vi "AH 2700 Single Measurement.vi"() -> ()   [LabVIEW 2019]
doc: "This example shows how to configure the bridge, take a single capacitance measurement, read the results from the bridge, and parse the measurement results."
uses:
  Andeen-Hagerling 2700(400 firmware).lvlib
panel:
  out "Loss Greater Than":string
  out "Attentap":string
  out "Sample Switch":i32
  out "Frequency (Hz)":dbl
  out "Result Units":i32(ring)=1 items=["nanosiemens"=1, "dissipation factor"=2, "kilohms"=3, "gigohms"=4, "loss vector (jpF)"=5]
  out "Error Message":string
  out "Voltage (V)":dbl format="%#_6f"
  out "Loss":dbl
  out "Capacitance (pF)":dbl format="%#_10f"
  in  "Units":i32(ring)=1 items=["nanosiemens"=1, "dissipation factor"=2, "kilohms"=3, "gigohms"=4, "loss vector (jpF)"=5]
  in  "Bridge Frequency (Hz)":dbl(ring)=1000.0 items=["50"=50.0, "60"=60.0, "70"=70.0, "80"=80.0, "100"=100.0, "120"=120.0, "140"=140.0, "160"=160.0, "200"=200.0, "240"=240.0, "300"=300.0, "400"=400.0, "500"=500.0, "600"=600.0, "700"=700.0, "800"=800.0, "1000"=1000.0, "1200"=1200.0, "1400"=1400.0, "1600"=1600.0, "2000"=2000.0, "2400"=2400.0, "3000"=3000.0, "4000"=4000.0, "5000"=5000.0, "6000"=6000.0, "7000"=7000.0, "8000"=8000.0, "10000"=10000.0, "12000"=12000.0, "14000"=14000.0, "16000"=16000.0, "20000"=20000.0]
  in  "Maximum Voltage (V)":dbl=15.0 min=0.0003 max=15.0 step=1.0 format="%#.6f"
  in  "Average Exponent":u16=4 max=15
  in  "VISA Resource":refnum<visa-resource-name>
  in  "Serial Configuration":T1={"Baud Rate"=9600, "Parity"=0, "Data Bits"=8, "Stop Bits"=10} {"Stop Bits" items=["1.0"=10, "1.5"=15, "2.0"=20]; "Data Bits" items=["7"=7, "8"=8]; "Parity" items=["None", "Odd", "Even", "Mark", "Space"]; "Baud Rate" items=["300"=300, "600"=600, "1200"=1200, "2400"=2400, "4800"=4800, "9600"=9600, "19200"=19200]}
  # "AH 2700A ULTRA-PRECISION 50Hz-20kHz CAPACITANCE BRIDGE"
  # "Single Measurement"
  # "Measurement Parameters"
  # "Measurement Results"
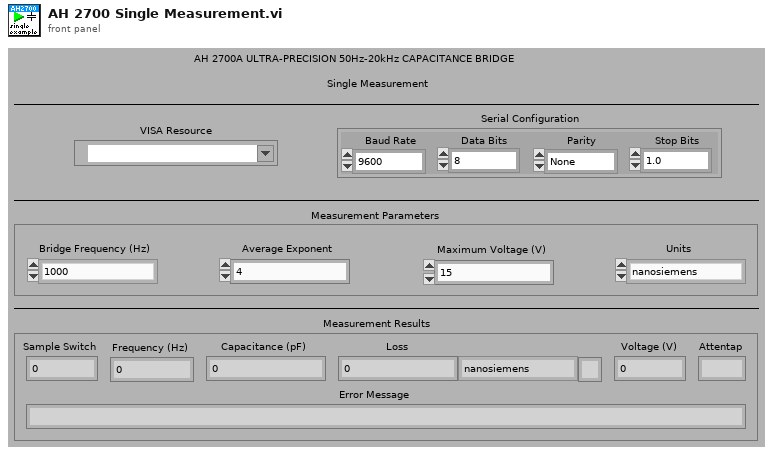
[diagram p1: front panel]
types:
  T1 = cluster{"Baud Rate":u32, "Parity":u16, "Data Bits":u16, "Stop Bits":u16}
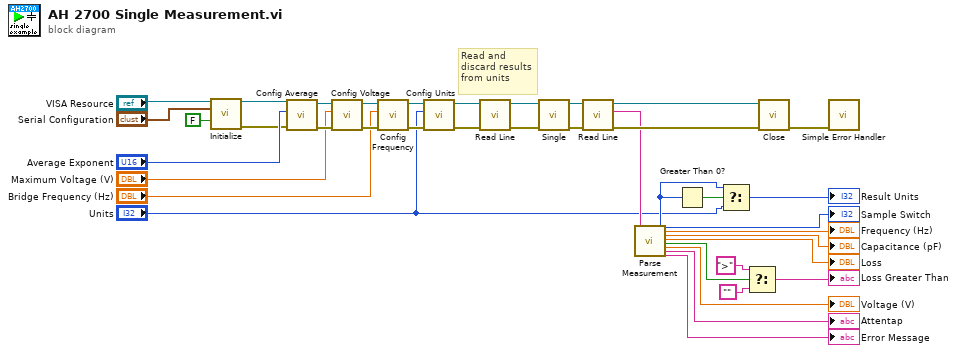
[diagram p0: block diagram]
diagram:
  # "Read and\ndiscard results\nfrom units"
  n1 = call "Initialize.vi"("VISA resource name"="VISA Resource", "Serial Configuration"="Serial Configuration", "Reset (True)"=FALSE) -> ("VISA resource name out"=w20:refnum<visa-resource-name>, "error out"=w21:errorcluster)  [unwired: 11 in]
  n2 = call "Config Average.vi"("error in"=w21, "Average Exponent (4)"="Average Exponent", "VISA resource name"=w20) -> ("error out"=w36:errorcluster, "VISA resource name out"=w39:refnum<visa-resource-name>)  [unwired: 7 in]
  n3 = call "Config Voltage.vi"("error in"=w36, "Voltage (15 V)"="Maximum Voltage (V)", "VISA resource name"=w39) -> ("error out"=w35:errorcluster, "VISA resource name out"=w38:refnum<visa-resource-name>)  [unwired: 7 in]
  n4 = call "Config Frequency.vi"("error in"=w35, "Frequency (1000 Hz)"="Bridge Frequency (Hz)", "VISA resource name"=w38) -> ("error out"=w34:errorcluster, "VISA resource name out"=w37:refnum<visa-resource-name>)  [unwired: 7 in]
  n5 = call "Config Units.vi"("error in"=w34, "Units (nS)"="Units", "VISA resource name"=w37) -> ("error out"=w29:errorcluster, "VISA resource name out"=w30:refnum<visa-resource-name>)  [unwired: 7 in]
  n6 = call "Read Line.vi"("error in"=w29, "VISA resource name"=w30) -> ("error out"=w27:errorcluster, "VISA resource name out"=w28:refnum<visa-resource-name>)  [unwired: 6 in, 2 out]
  n7 = call "Single.vi"("error in"=w27, "VISA resource name"=w28) -> ("error out"=w25:errorcluster, "VISA resource name out"=w26:refnum<visa-resource-name>)  [unwired: 8 in]
  n8 = call "Read Line.vi"("error in"=w25, "VISA resource name"=w26) -> ("error out"=w23:errorcluster, "Message"=w16:string, "VISA resource name out"=w24:refnum<visa-resource-name>)  [unwired: 6 in, 1 out]
  n9 = call "Parse Measurement.vi"("Measurement Line"=w16) -> ("Units"=w6:i32, "Sample"=→"Sample Switch":i32, "Frequency"=→"Frequency (Hz)":dbl, "Capacitance"=→"Capacitance (pF)":dbl, "Loss"=→"Loss":dbl, "Loss Greater Than"=w11:bool, "Voltage"=→"Voltage (V)":dbl, "Attentap"=→"Attentap":string, "Error Message"=→"Error Message":string)  [unwired: 17 in, 1 out]
  n10 = Greater Than 0?(x=w6) -> (x > 0?=w7:bool)
  n11 = Select(t=w6, s=w7, f="Units") -> (s? t:f=→"Result Units":i32)
  n12 = Select(t=">", s=w11, f="") -> (s? t:f=→"Loss Greater Than":string)
  n13 = call "Close.vi"("error in (no error)"=w23, "VISA resource name"=w24) -> ("error out"=w22:errorcluster)  [unwired: 9 in]
  n14 = call <vilib>:"Simple Error Handler.vi"("error in (no error)"=w22) -> ()  [unwired: 4 in, 5 out]
